vi "MDF4 Create Data Group.vi"(7 "path in":path, 8 "Error In":errorcluster, 11 "MDF4 File Reference in":i64) -> (0 "Error Out":errorcluster, 2 "Data Group Reference out":i64, 3 "MDF4 File Reference out":i64)   [LabVIEW 2019, in "MD4Logger Engine.lvlib"]
uses:
  MD4Logger Engine.lvlib
  <vilib>/Utility/error.llb/Error Cluster From Error Code.vi
  <vilib>/ErrorRing/Error Ring.xnode
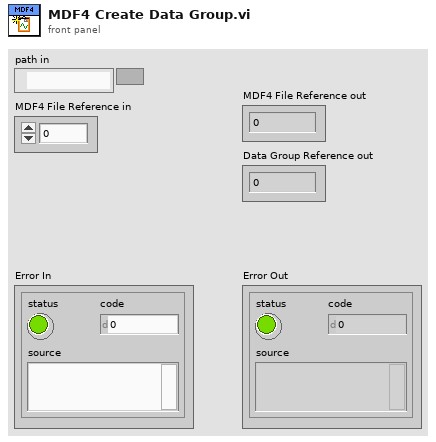
[diagram p1: front panel]
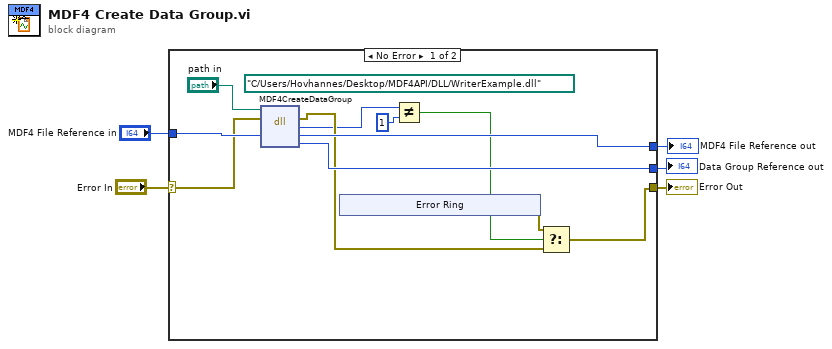
[diagram p0: block diagram]
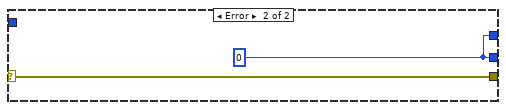
[diagram p2: hidden frame]
diagram:
  n1 = case shown="No Error" "Error In" {
    selector: "Error In" -> [w15 w23]
    tunnel: "MDF4 File Reference in" -> [w16 _]
    tunnel: [w10 w23] -> w3
    tunnel: [w14 w22] -> w2
    tunnel: [w13 w22] -> w1
    frame No Error {
      (unwired) path "C:/Users/Hovhannes/Desktop/MDF4API/DLL/WriterExample.dll" ("path in")
      n2 = dll-call lib="C:/Users/Hovhannes/Desktop/MD4Logger/Source/Engine/DLL/WriterExample.dll" fn="MDF4CreateDataGroup"(path in="path in", error in=w15, "m4"=w16) -> (error out=w11:errorcluster, "return type"=w8:i32, "m4"=w13:i64, "dg"=w14:i64)  [unwired: 2 in, 1 out]
      n3 = xnode "Error Ring"() -> ("error out"=w12:errorcluster)
      n4 = Not Equal?(x=w8, y=1) -> (x != y?=w7:bool)
      n5 = Select(t=w12, s=w7, f=w11) -> (s? t:f=w10:errorcluster)
    }
    frame Error {
      w22 = i64 0 ("m4")
    }
  }
  "Data Group Reference out" <- w2
  "Error Out" <- w3
  "MDF4 File Reference out" <- w1
